vi "DifineDivergenceAngleAxisPos.vi"(4 "远场横向坐标队列":refnum<queue>, 5 "发散角横向坐标队列":refnum<queue>, 6 "发散角轴向坐标队列":refnum<queue>, 7 "位置":T1) -> ()   [LabVIEW 2018]
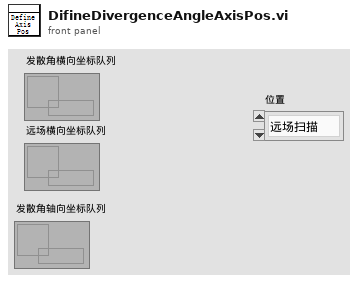
[diagram p1: front panel]
types:
  T1 = typedef "控制电机位置枚举器.ctl" = enum16{"远场扫描", "发散角扫描", "远场相机", "近场相机", "时间波形", "偏振", "能量", "功率", "光谱"}
  T2 = typedef "控制电机枚举器.ctl" = enum16{"Z", "Y", "X", "发散角", "俯仰", "旋转"}
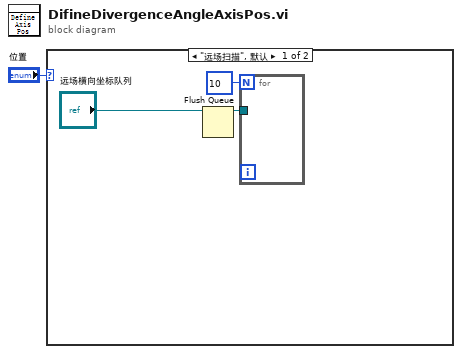
[diagram p0: block diagram]
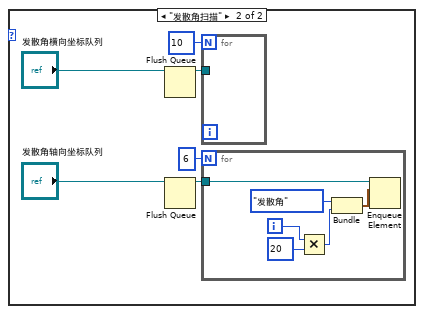
[diagram p2: hidden frame]
diagram:
  n1 = case shown="\"远场扫描\", 默认" "位置" {
    frame "远场扫描", Default {
      n2 = Flush Queue(queue="远场横向坐标队列") -> (queue out=w3:refnum<queue>)  [unwired: 1 in, 2 out]
      n3 = for {
        N: 10 -> [_]
        tunnel: w3 -> [_]
      }
    }
    frame "发散角扫描" {
      n4 = Flush Queue(queue="发散角横向坐标队列") -> (queue out=w6:refnum<queue>)  [unwired: 1 in, 2 out]
      n5 = Flush Queue(queue="发散角轴向坐标队列") -> (queue out=w10:refnum<queue>)  [unwired: 1 in, 2 out]
      n6 = for {
        N: 10 -> [_]
        tunnel: w6 -> [_]
      }
      n7 = for {
        N: 6 -> [_]
        tunnel: w10 -> [w16]
        i -> [w15]
        n8 = Multiply(x=w15, y=20) -> (x*y=w12:i32)
        n9 = Bundle("控制电机"=控制电机枚举器."发散角", w12) -> (w11:cluster{"控制电机":T2, i32})  [unwired: 1 in]
        n10 = Enqueue Element(queue=w16, element=w11) -> ()  [unwired: 2 in, 3 out]
      }
    }
  }
